vi "纳清浊度电极校准.vi"() -> ()   [LabVIEW 2016, in "斯坦道多参数.lvlib"]
uses:
  <vilib>/Utility/miscctls.llb/LVPointTypeDef.ctl
  <vilib>/Utility/miscctls.llb/LVPositionTypeDef.ctl
  <vilib>/Analysis/NI_AALBase.lvlib
  <vilib>/ptbypt/NI_PtbyPt.lvlib
panel:
  out "第三点信号值":dbl
  out "第二点信号值":dbl
  out "第一点信号值":dbl
  in  "校准量程":u16(ring) items=["0-100", "0-500", "0-2000", "0-4000"]
  in  "量程":u16(ring) items=["0-100", "0-500", "0-2000", "0-4000"]
  out "报警信息":string
  out "通讯状态":string
  out "第三点校准值":dbl
  out "标液3":sgl
  out "第二点校准值":dbl
  out "第一点校准值":dbl
  in  "校准停止":bool
  in  "校准启动":bool
  in  "校准模式":enum16{"两点校准", "单点校准", "三点校准"}(ring)=enum."单点校准"
  out "最小值":sgl format="%#.2f"
  out "最大值":sgl format="%#.2f"
  out "波形图表":dbl(graph) caption="历史曲线"
  out "mean":dbl caption="均值" format="%#.2f"
  out "standard deviation":dbl caption="标准差" format="%#.2f"
  out "变异系数":dbl format="%#.6f"
  out "测量值":sgl format="%#.2f"
  out "提示":string
  out "标液2":sgl
  out "标液1":sgl
  out "原始光强数值":u16 caption="信号值"
  out "温度":dbl format="%#.2f"
  # "浊度电极设定"
  # "℃"
  # "NTU"
  # "NTU"
  # "NTU"
  # "请选择校准模式:"
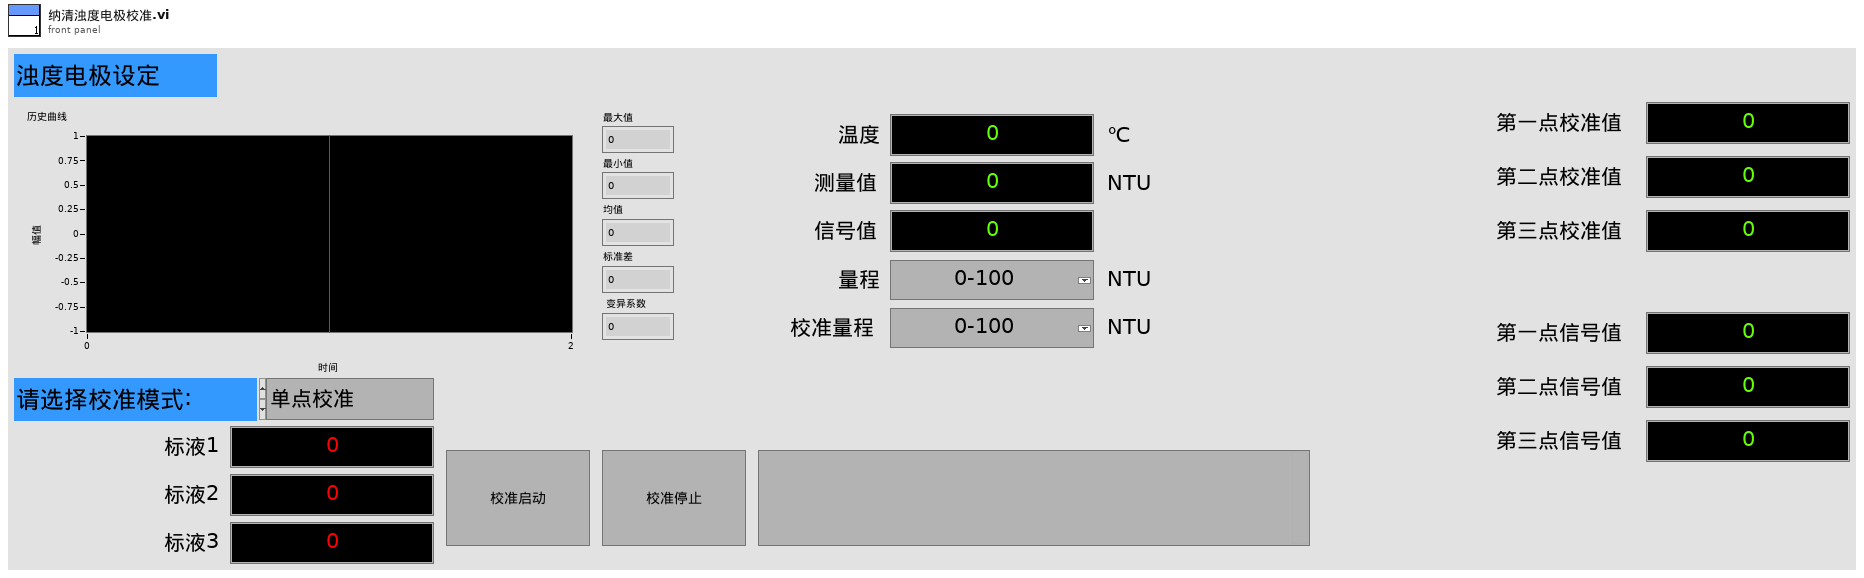
[diagram p1: front panel]
types:
  T1 = typedef "LVPointTypeDef.ctl" = cluster{"Horizontal":i16, "Vertical":i16}
  T2 = cluster{"报警码":u16, "浊度数值 NTU":sgl, "温度数据":sgl, "原始光强数值":u16, "量程":u16, "平均次数":u16, "清扫模式":u16, "清扫次数":u16, "清扫间隔分钟":u16, "0X000B_NC":string, "产品名称":string, "序列号":string, "硬件版本":string, "软件版本":string, "通讯地址":u16, "波特率":u16, "设备类型":u16, "0X0026_NC":string, "校准量程":u16, "第一点原始光强":u16, "第一点校准数据":sgl, "第二点原始光强":u16, "第二点校准数据":sgl, "第三点原始光强":u16, "第三点校准数据":sgl, "探头校准命令":u16, "温度校准参数":sgl, "温度校准命令":u16}
  T3 = typedef "LVPositionTypeDef.ctl" = cluster{"Left":i32, "Top":i32}
  T4 = enum8{"Enabled", "Disabled", "Disabled and Grayed Out"}
  T5 = cluster{"报警码":u16, "叶绿素a":sgl, "温度数据":sgl, "原始光强数值":u16, "量程":u16, "平均次数":u16, "清扫模式":u16, "清扫次数":u16, "清扫间隔分钟":u16, "0X000B_NC":string, "产品名称":string, "序列号":string, "硬件版本":string, "软件版本":string, "通讯地址":u16, "波特率":u16, "设备类型":u16, "0X0026_NC":string, "校准量程":u16, "第一点原始光强":u16, "第一点校准数据":sgl, "第二点原始光强":u16, "第二点校准数据":sgl, "第三点原始光强":u16, "第三点校准数据":sgl, "探头校准命令":u16, "温度校准参数":sgl, "温度校准命令":u16}
  T6 = cluster{"ph":bool, "DO":bool, "Cond":bool, "Turb":bool, "叶绿素a":bool, "藻密度":bool, "ORP":bool}
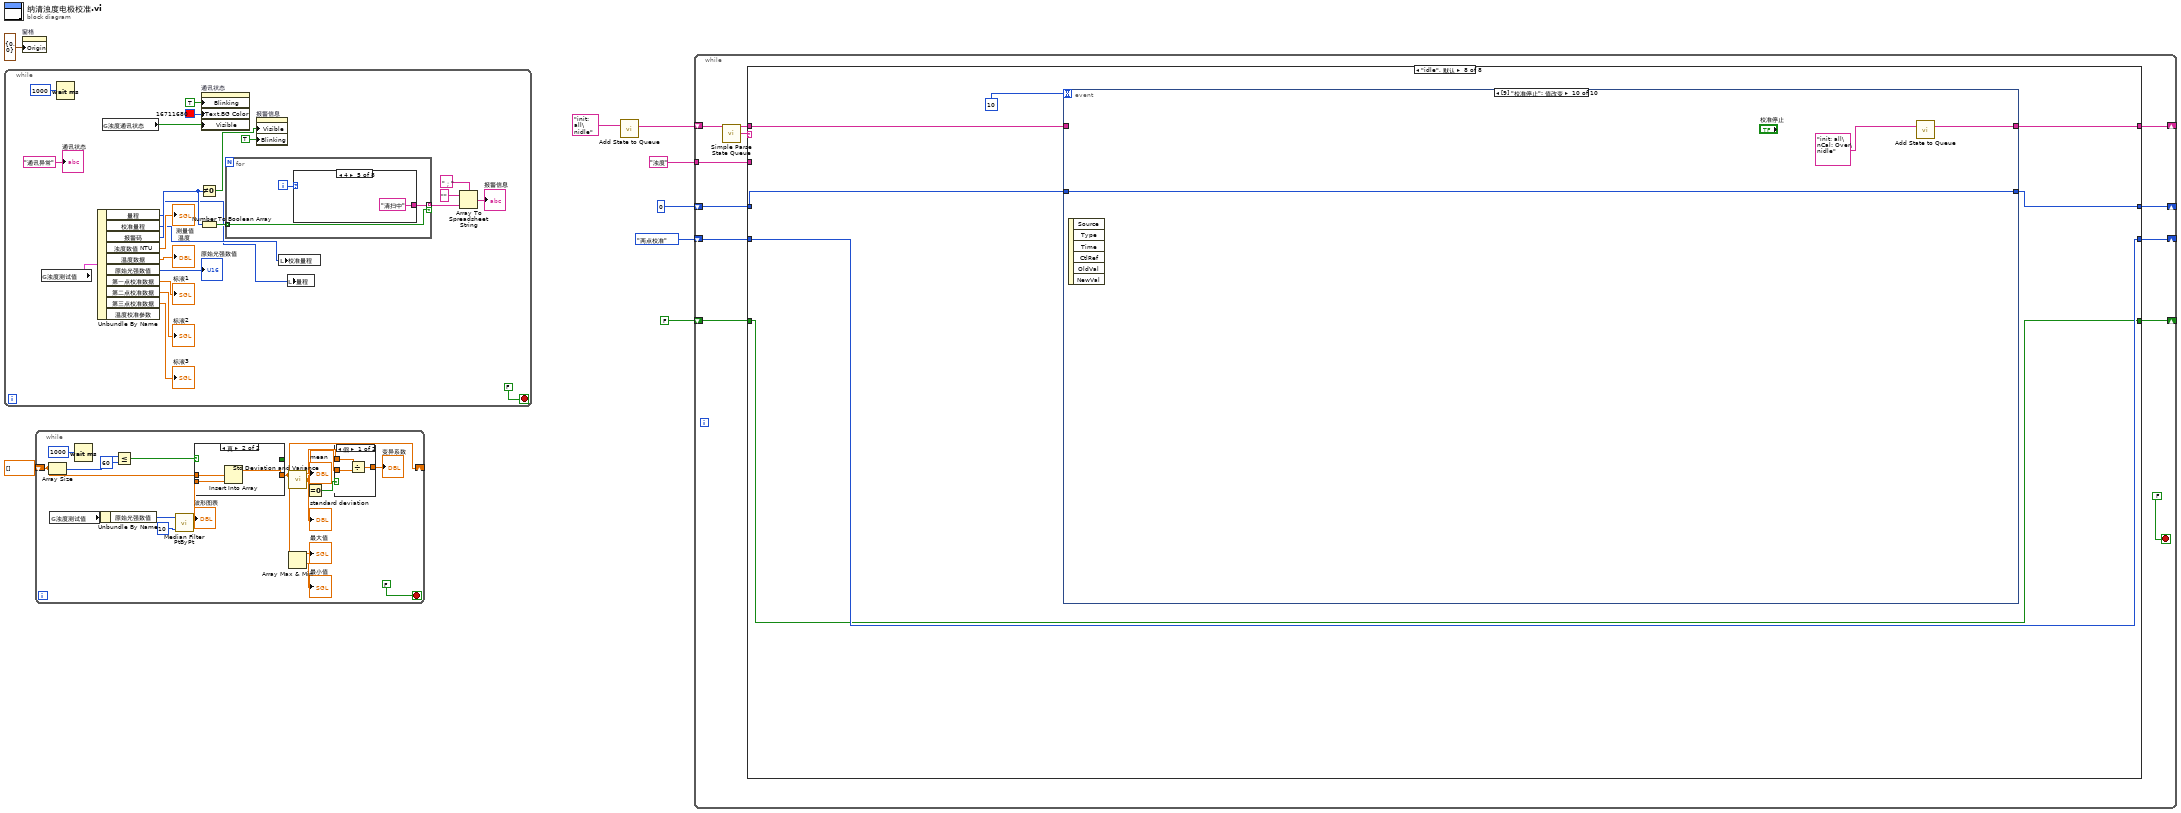
[diagram p0: block diagram]
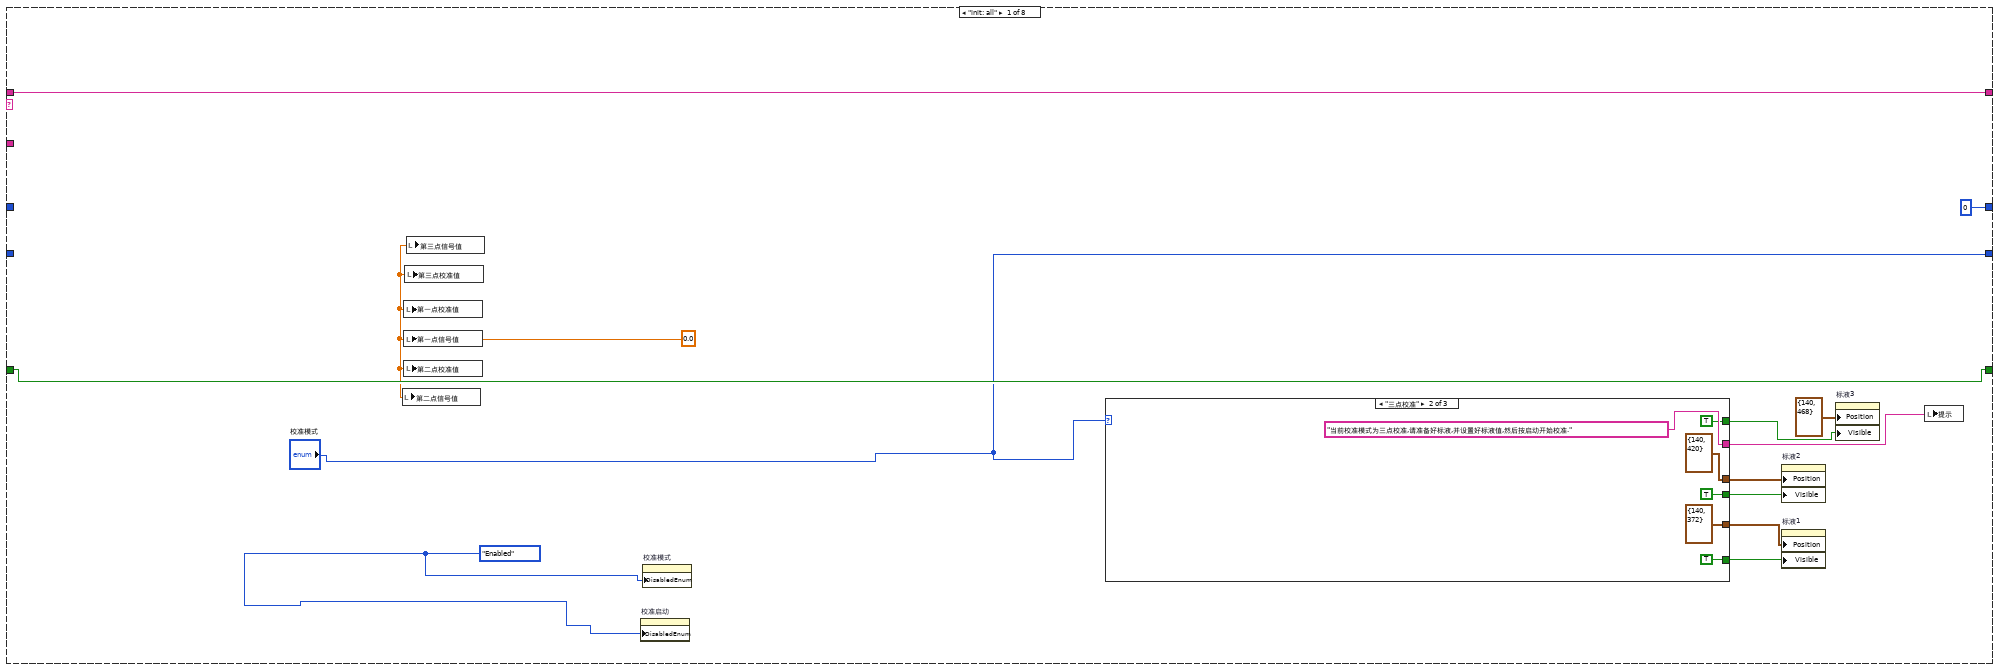
[diagram p2: hidden frame]
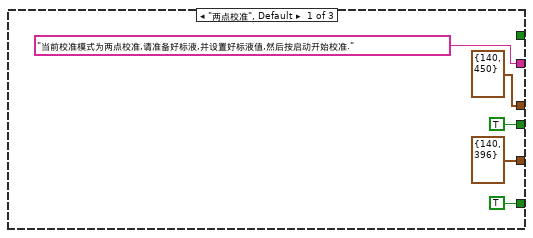
[diagram p3: hidden frame]
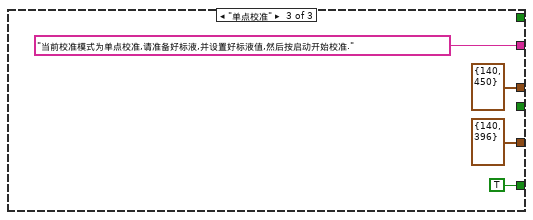
[diagram p4: hidden frame]
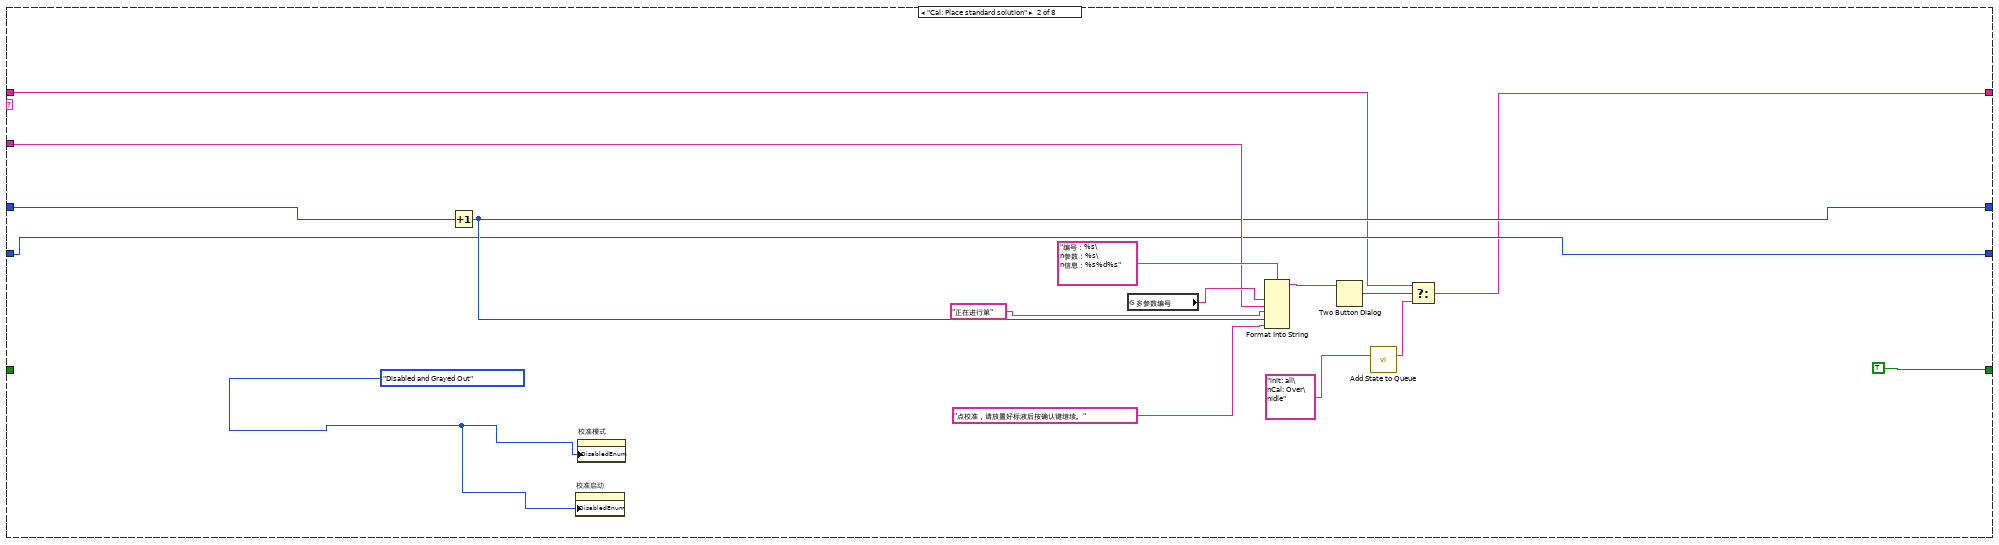
[diagram p5: hidden frame]
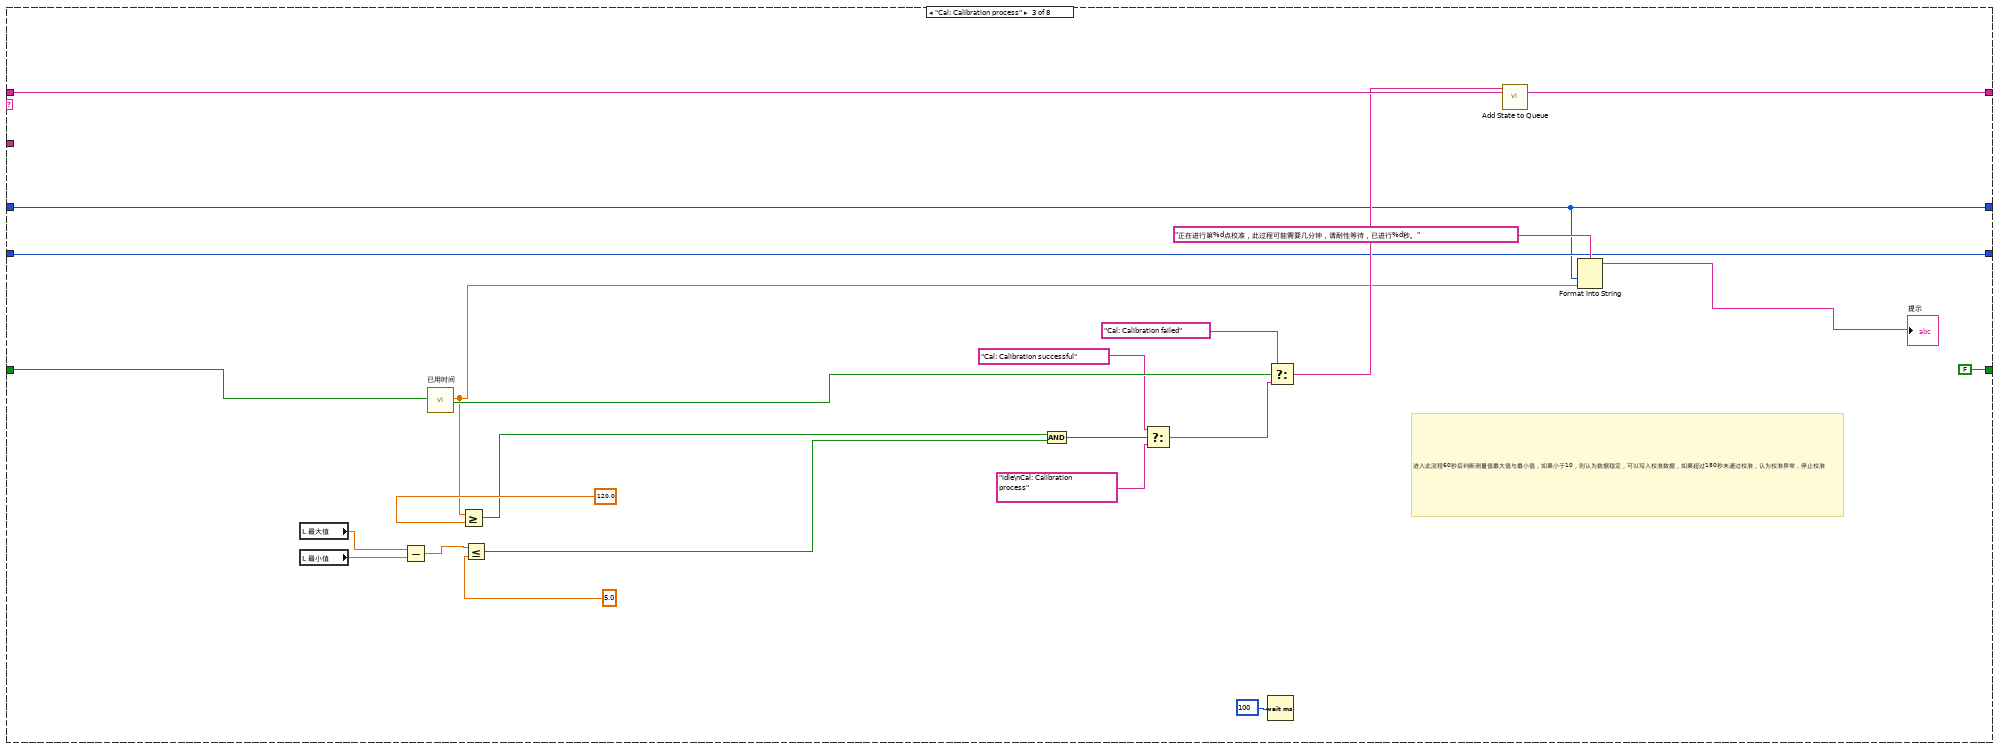
[diagram p6: hidden frame]
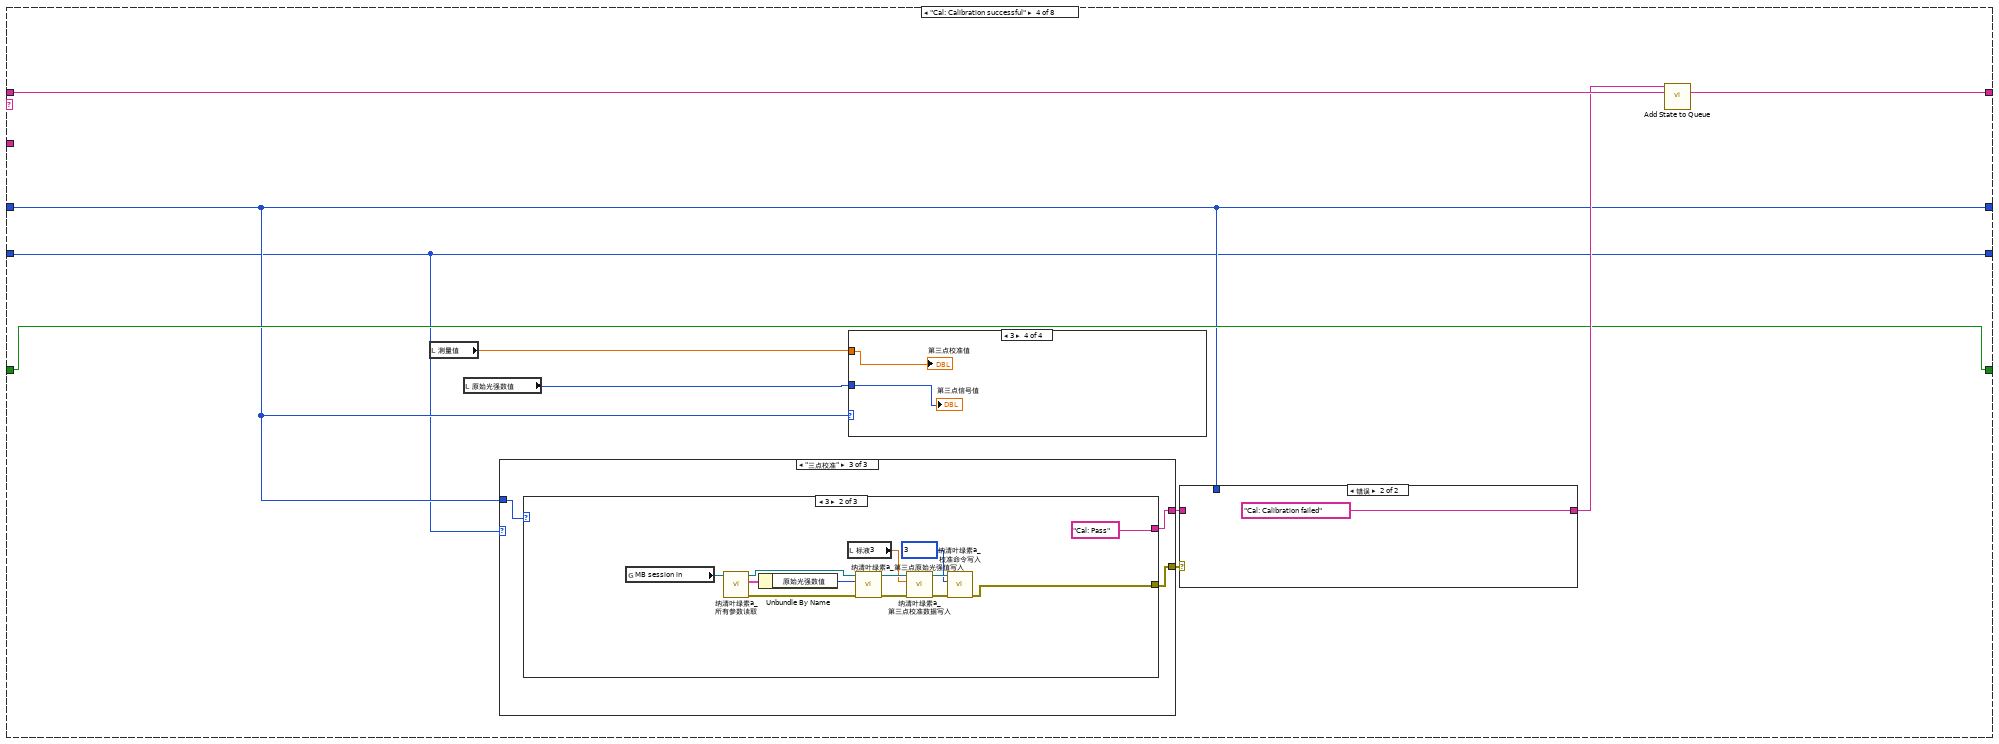
[diagram p7: hidden frame]
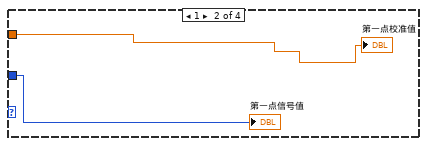
[diagram p9: hidden frame]
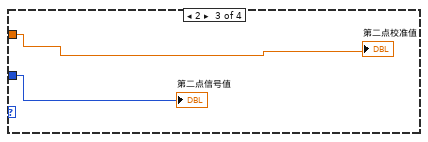
[diagram p10: hidden frame]
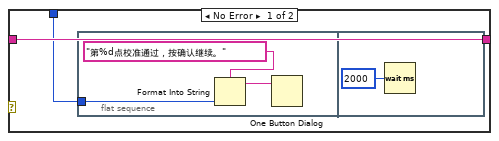
[diagram p11: hidden frame]
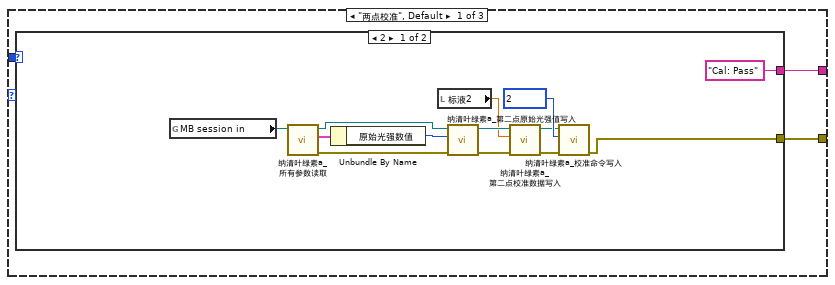
[diagram p12: hidden frame]
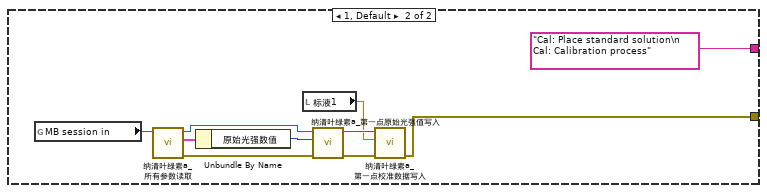
[diagram p13: hidden frame]
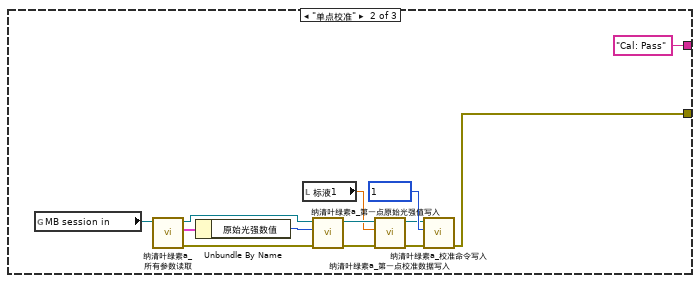
[diagram p14: hidden frame]
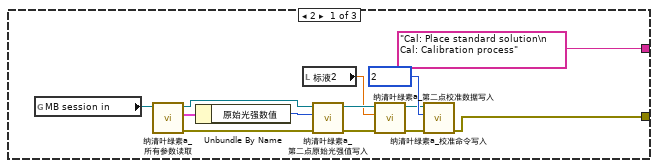
[diagram p15: hidden frame]
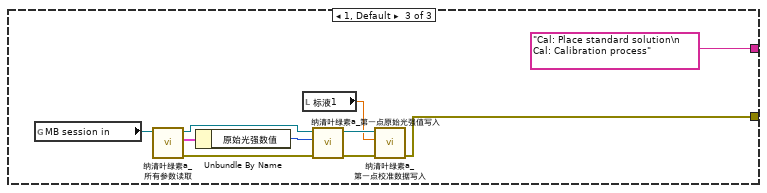
[diagram p16: hidden frame]
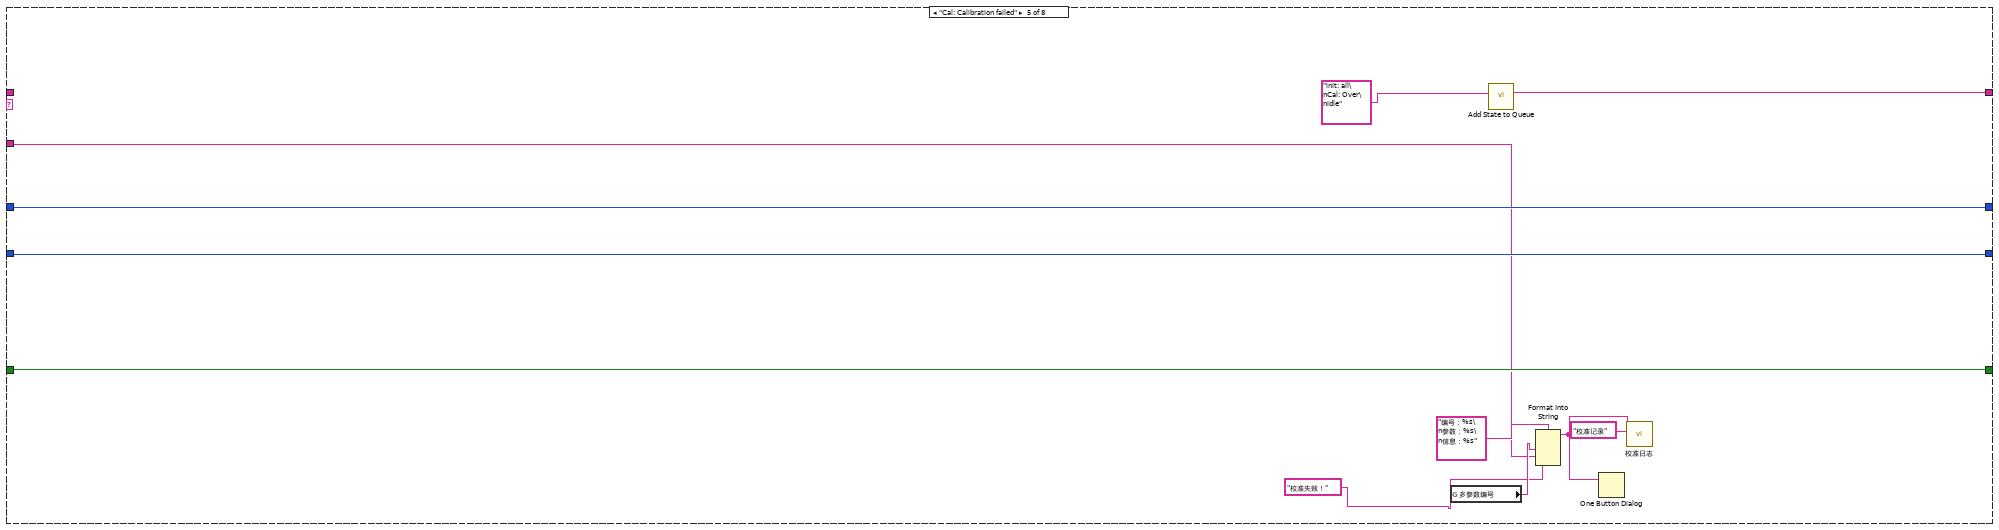
[diagram p17: hidden frame]
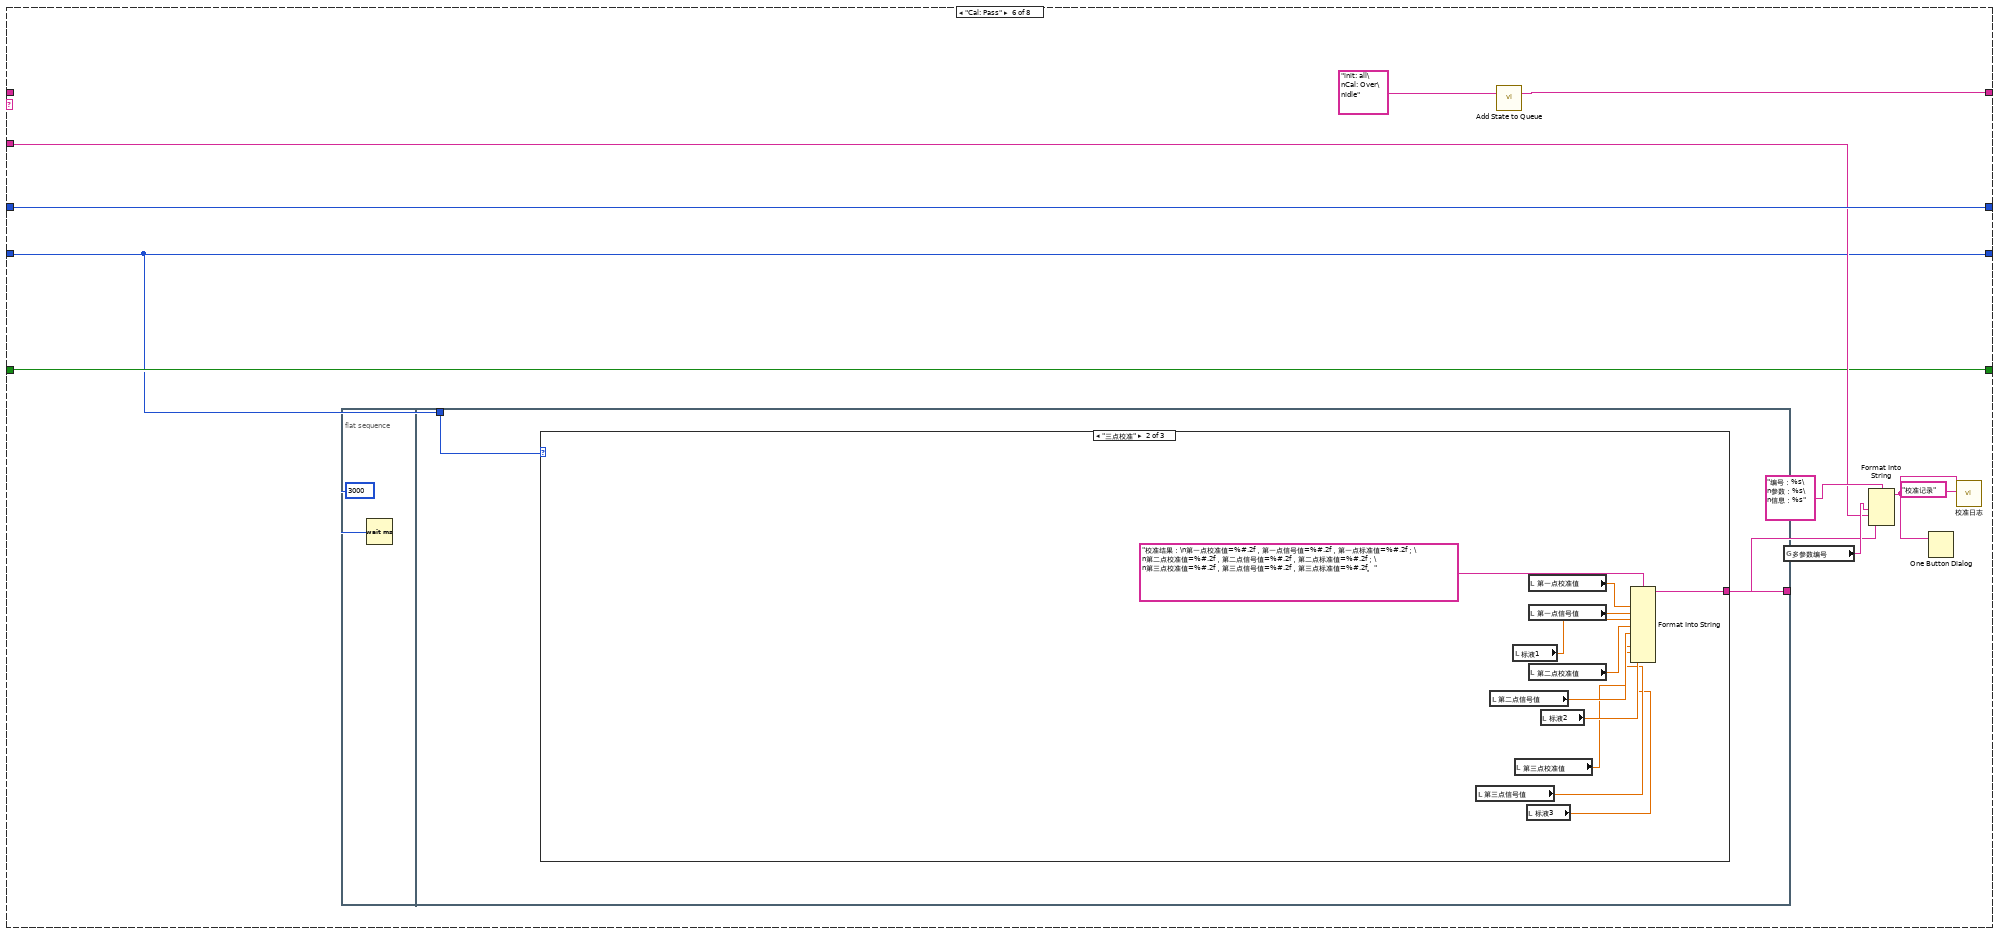
[diagram p18: hidden frame]
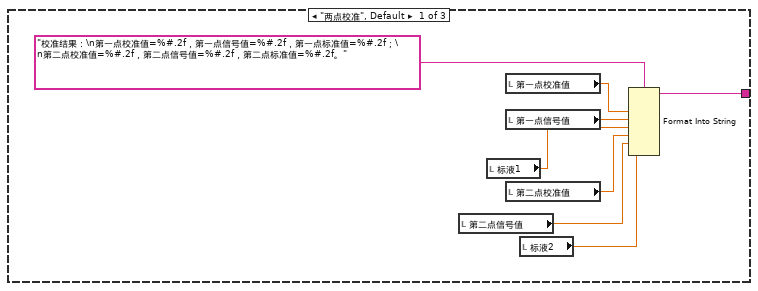
[diagram p19: hidden frame]
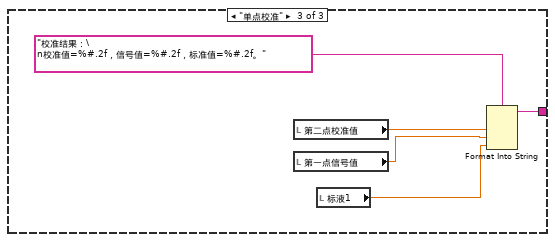
[diagram p20: hidden frame]
diagram:
  n1 = while {
    stop <- FALSE stop-if-true
    n2 = global read "纳清过程全局变量.vi" "浊度测试值"() -> (w29:T2)
    n3 = Wait (ms)(milliseconds to wait=u32 1000 ("等待时间（毫秒）")) -> ()  [unwired: 1 out]
    n4 = Unbundle By Name(w29) -> ("量程"=w9:u16, "校准量程"=w10:u16, "报警码"=w11:u16, "浊度数值 NTU"=→"测量值":sgl, "温度数据"=→"温度":sgl, "原始光强数值"=→"原始光强数值":u16, "第一点校准数据"=→"标液1":sgl, "第二点校准数据"=→"标液2":sgl, "第三点校准数据"=→"标液3":sgl)  [unwired: 1 out]
    n5 = global read "多参数全局变量.vi" "浊度通讯状态"() -> (w19:bool)
    n6 = Not Equal To 0?(x=w11) -> (x != 0?=w13:bool)
    n7 = Number To Boolean Array(number=w11) -> (Boolean array=w18:bool[])
    n8 = property on="通讯状态" class="Str"("Blinking"=TRUE ("闪烁"), "Text.BG Color"=u32 16711680, "Visible"=w19) -> ()  [unwired: 2 in, 2 out]
    n9 = for {
      tunnel: w18 -> [w32] mode=indexing
      tunnel: [w33] -> w17 mode=indexing if=w32
      i -> [w34]
      n10 = case shown="4" w34 {
        tunnel: [_ "浊度超量程" "温度超量程" "光强信号超范围" "清扫中" "温度传感器故障" "电极故障" "内部电压基准故障"] -> w33
        frame Default {
        }
        frame 0 {
        }
        frame 2 {
        }
        frame 3 {
        }
        frame 4 {
        }
        frame 8 {
        }
        frame 9 {
        }
        frame 10 {
        }
      }
    }
    n11 = property on="报警信息" class="Str"("Visible"=w13, "Blinking"=TRUE ("闪烁")) -> ()  [unwired: 2 in, 2 out]
    n12 = local write "校准量程"(w10) -> ()
    n13 = local write "量程"(w9) -> ()
    n14 = Array To Spreadsheet String(delimiter (Tab)="；" ("分隔符(Tab)"), array=w17, 3:"" ("格式字符串")) -> (spreadsheet string=→"报警信息":string)
    "通讯状态" <- "通讯异常" ("当前串口")
  }
  n15 = property on="窗格" class="Pane"("Origin"=T1 {"Horizontal"=0, "Vertical"=0} ("原点")) -> ()  [unwired: 2 in, 2 out]
  n16 = while {
    shift-right: [w48] -> _
    shift-left: sgl[] [] -> [w54]
    stop <- FALSE stop-if-true
    n17 = Array Size(array=w54) -> (size(s)=w56:i32)
    n18 = global read "纳清过程全局变量.vi" "浊度测试值"() -> (w45:T2)
    n19 = Wait (ms)(milliseconds to wait=u32 1000 ("等待时间（毫秒）")) -> ()  [unwired: 1 out]
    n20 = Unbundle By Name(w45) -> ("原始光强数值"=w43:u16)
    n21 = Less Or Equal?(x=w56, y=60) -> (x <= y?=w55:bool)
    n22 = call <vilib>:"Median Filter PtByPt.vi"("rank"=10, "x"=w43) -> ("Filtered x"=w42:dbl)  [unwired: 2 in, 1 out]
    "波形图表" <- w42
    n23 = case shown="真" w55 {
      tunnel: w54 -> [w67 w70]
      tunnel: w42 -> [w65 w69]
      tunnel: [w63 w68] -> w48
      tunnel: [TRUE _] -> _
      frame False {
        n24 = Replace Array Subset(array=w67, new element=w65) -> (w66:sgl[])  [unwired: 1 in]
        n25 = Rotate 1D Array(1:w66, 2:-1 ("n")) -> (0:w63:sgl[])
      }
      frame True {
        n26 = Insert Into Array(array=w70, new element=w69) -> (w68:sgl[])  [unwired: 1 in]
      }
    }
    n27 = call <vilib>:"Std Deviation and Variance.vi"("X"=w48) -> ("mean"=w52:dbl, "standard deviation"=w51:dbl)  [unwired: 1 in, 1 out]
    "mean" <- w52
    "standard deviation" <- w51
    n28 = Array Max & Min(array=w48) -> (max value=→"最大值":sgl, min value=→"最小值":sgl)  [unwired: 2 out]
    n29 = Equal To 0?(x=w52) -> (x = 0?=w53:bool)
    n30 = case shown="假" w53 {
      tunnel: w51 -> [w61 _]
      tunnel: [w60 _] -> w50
      tunnel: w52 -> [w59 _]
      frame False {
        n31 = Divide(x=w61, y=w59) -> (x/y=w60:dbl)
      }
      frame True {
      }
    }
    "变异系数" <- w50
  }
  n32 = call "Add State to Queue.vi"("State(s) In (\"\")"="init: all\nidle" ("State(s) In (\"\")")) -> ("States Out"=w5:string)  [unwired: 14 in]
  n33 = while {
    shift-right: [w78] -> _
    shift-left: w5 -> [w82]
    shift-right: [w75] -> _
    shift-left: 0 -> [w77]
    tunnel: "浊度" ("State(s) In (\"\")") -> [w76]
    shift-right: [w73] -> _
    shift-left: enum16{"两点校准", "单点校准", "三点校准"}."两点校准" ("校准模式") -> [w74]
    shift-right: [w71] -> _
    shift-left: FALSE -> [w72]
    stop <- FALSE stop-if-true
    n34 = call "Simple Parse State Queue.vi"("State Queue"=w82) -> ("Remain States"=w79:string, "Next State"=w80:string)  [unwired: 13 in]
    n35 = case shown="\"idle\", 默认" w80 {
      tunnel: w79 -> [w95 w114 w145 w158 _ _ w307 w314]
      tunnel: [w95 w113 w144 w157 w259 w264 w307 w313] -> w78
      tunnel: w77 -> [_ w122 w129 w152 w262 w273 w306 w311]
      tunnel: w76 -> [_ w123 _ _ w253 w269 _ _]
      tunnel: [0 w120 w129 w152 w262 w273 w306 w312] -> w75
      tunnel: w74 -> [_ w119 w130 w151 w261 w265 w305 w310]
      tunnel: ["校准模式" w119 w130 w151 w261 w265 w305 w310] -> w73
      tunnel: w72 -> [w93 _ w132 w153 w260 w268 w304 w308]
      tunnel: [w93 TRUE FALSE w153 w260 w268 w304 w308] -> w71
      frame "init: all" {
        w91 = T4."Enabled" ("禁用")
        w92 = 0.0 ("第一点校准值")
        n36 = local write "第二点信号值"(w92) -> ()
        n37 = local write "第一点校准值"(w92) -> ()
        n38 = local write "第一点信号值"(w92) -> ()
        n39 = local write "第二点校准值"(w92) -> ()
        n40 = local write "第三点校准值"(w92) -> ()
        n41 = local write "第三点信号值"(w92) -> ()
        n42 = property on="校准启动" class="Bool"("DisabledEnum"=w91) -> ()  [unwired: 2 in, 2 out]
        n43 = property on="校准模式" class="Enum (严格)"("DisabledEnum"=w91) -> ()  [unwired: 2 in, 2 out]
        n44 = case shown="\"三点校准\"" "校准模式" {
          tunnel: ["当前校准模式为两点校准,请准备好标液,并设置好标液值,然后按启动开始校准." ("提示") "当前校准模式为三点校准,请准备好标液,并设置好标液值,然后按启动开始校准." ("提示") "当前校准模式为单点校准,请准备好标液,并设置好标液值,然后按启动开始校准." ("提示")] -> w83
          tunnel: [TRUE ("可见") TRUE ("可见") _] -> w88
          tunnel: [T3 {"Left"=140, "Top"=396} ("位置") T3 {"Left"=140, "Top"=372} ("位置") T3 {"Left"=140, "Top"=396} ("位置")] -> w85
          tunnel: [T3 {"Left"=140, "Top"=450} ("位置 2") T3 {"Left"=140, "Top"=420} ("位置 2") T3 {"Left"=140, "Top"=450} ("位置 2")] -> w86
          tunnel: [_ TRUE ("可见") _] -> w89
          tunnel: [TRUE ("可见") TRUE ("可见") TRUE ("可见")] -> w90
          frame "两点校准", Default {
          }
          frame "三点校准" {
          }
          frame "单点校准" {
          }
        }
        n45 = property on="标液2" class="DigNum (严格)"("Position"=w86, "Visible"=w88) -> ()  [unwired: 2 in, 2 out]
        n46 = property on="标液1" class="DigNum (严格)"("Position"=w85, "Visible"=w90) -> ()  [unwired: 2 in, 2 out]
        n47 = property on="标液3" class="DigNum (严格)"("Position"=T3 {"Left"=140, "Top"=468} ("位置 3"), "Visible"=w89) -> ()  [unwired: 2 in, 2 out]
        n48 = local write "提示"(w83) -> ()
      }
      frame "Cal: Place standard solution" {
        w112 = T4."Disabled and Grayed Out" ("禁用")
        n49 = Increment(x=w122) -> (x+1=w120:i32)
        n50 = property on="校准启动" class="Bool"("DisabledEnum"=w112) -> ()  [unwired: 2 in, 2 out]
        n51 = property on="校准模式" class="Enum (严格)"("DisabledEnum"=w112) -> ()  [unwired: 2 in, 2 out]
        n52 = global read "多参数全局变量.vi" "多参数编号"() -> (w125:string)
        n53 = Format Into String(format string="编号：%s\n参数：%s\n信息：%s%d%s" ("格式字符串"), w125, w123, "正在进行第" ("消息"), w120, "点校准，请放置好标液后按确认键继续。" ("消息")) -> (resulting string=w117:string)  [unwired: 2 in, 1 out]
        n54 = Two Button Dialog(message=w117) -> (T button?=w116:bool)  [unwired: 2 in]
        n55 = call "Add State to Queue.vi"("State(s) In (\"\")"="init: all\nCal: Over\nidle" ("State(s) In (\"\")")) -> ("States Out"=w115:string)  [unwired: 14 in]
        n56 = Select(t=w114, s=w116, f=w115) -> (s? t:f=w113:string)
      }
      frame "Cal: Calibration process" {
        # "进入此流程60秒后判断测量值最大值与最小值，如果小于10，则认为数据稳定，可以写入校准数据，如果超过180秒未通过校准，认为校准异常，停止校准"
        n57 = local read "最大值"() -> (w149:sgl)
        n58 = local read "最小值"() -> (w148:sgl)
        n59 = Subtract(x=w149, y=w148) -> (x-y=w150:sgl)
        n60 = call "已用时间"("Reset"=w132) -> ("Elapsed Time (s)"=w128:dbl, "Time has Elapsed"=w146:bool)  [unwired: 11 in, 6 out]
        n61 = Greater Or Equal?(x=w128, y=120.0) -> (x >= y?=w141:bool)
        n62 = Less Or Equal?(x=w150, y=5.0) -> (x <= y?=w137:bool)
        n63 = And(x=w141, y=w137) -> (x .and. y?=w138:bool)
        n64 = Select(t="Cal: Calibration successful" ("State(s) In (\"\")"), s=w138, f="idle\nCal: Calibration process" ("State(s) In (\"\")")) -> (s? t:f=w136:string)
        n65 = Wait (ms)(milliseconds to wait=u32 100 ("等待时间（毫秒）")) -> ()  [unwired: 1 out]
        n66 = Select(t="Cal: Calibration failed" ("State(s) In (\"\")"), s=w146, f=w136) -> (s? t:f=w135:string)
        n67 = call "Add State to Queue.vi"("State(s) In Front (\"\")"=w135, "State(s) In (\"\")"=w145) -> ("States Out"=w144:string)  [unwired: 13 in]
        n68 = Format Into String(format string="正在进行第%d点校准，此过程可能需要几分钟，请耐性等待，已进行%d秒。" ("格式字符串"), w129, w128) -> (resulting string=→"提示":string)  [unwired: 2 in, 1 out]
      }
      frame "Cal: Calibration successful" {
        n69 = local read "测量值"() -> (w154:sgl)
        n70 = local read "原始光强数值"() -> (w155:u16)
        n71 = case shown="\"三点校准\"" w151 {
          tunnel: [w176 w200 w213] -> w160
          tunnel: [w175 "Cal: Pass" ("State(s) In (\"\")") w214] -> w159
          tunnel: w152 -> [w174 _ w215]
          frame "两点校准", Default {
            n72 = case shown="2" w174 {
              tunnel: [w177 w190] -> w176
              tunnel: ["Cal: Pass" ("State(s) In (\"\")") "Cal: Place standard solution\n Cal: Calibration process" ("State(s) In (\"\")")] -> w175
              frame 2 {
                n73 = global read "多参数全局变量.vi" "MB session in"() -> (w185:refnum<class "MB_Master.lvclass">)
                n74 = call "纳清叶绿素a_所有参数读取.vi"("MB session in"=w185) -> ("error out"=w187:errorcluster, "输出值"=w184:T5, "MB session out"=w186:refnum<class "MB_Master.lvclass">)  [unwired: 8 in]
                n75 = Unbundle By Name(w184) -> ("原始光强数值"=w183:u16)
                n76 = local read "标液2"() -> (w178:sgl)
                n77 = call "纳清叶绿素a_第二点原始光强值写入.vi"("error in (no error)"=w187, "数值"=w183, "MB session in"=w186) -> ("error out"=w182:errorcluster, "MB session out"=w181:refnum<class "MB_Master.lvclass">)  [unwired: 7 in]
                n78 = call "纳清叶绿素a_第二点校准数据写入.vi"("error in (no error)"=w182, "数值"=w178, "MB session in"=w181) -> ("error out"=w180:errorcluster, "MB session out"=w179:refnum<class "MB_Master.lvclass">)  [unwired: 7 in]
                n79 = call "纳清叶绿素a_校准命令写入.vi"("error in (no error)"=w180, "数值"=u16 2 ("starting address"), "MB session in"=w179) -> ("error out"=w177:errorcluster)  [unwired: 7 in, 1 out]
              }
              frame 1, Default {
                n80 = global read "多参数全局变量.vi" "MB session in"() -> (w196:refnum<class "MB_Master.lvclass">)
                n81 = call "纳清叶绿素a_所有参数读取.vi"("MB session in"=w196) -> ("error out"=w198:errorcluster, "输出值"=w195:T5, "MB session out"=w197:refnum<class "MB_Master.lvclass">)  [unwired: 8 in]
                n82 = Unbundle By Name(w195) -> ("原始光强数值"=w194:u16)
                n83 = local read "标液1"() -> (w191:sgl)
                n84 = call "纳清叶绿素a_第一点原始光强值写入.vi"("error in (no error)"=w198, "数值"=w194, "MB session in"=w197) -> ("error out"=w193:errorcluster, "MB session out"=w192:refnum<class "MB_Master.lvclass">)  [unwired: 7 in]
                n85 = call "纳清叶绿素a_第一点校准数据写入.vi"("error in (no error)"=w193, "数值"=w191, "MB session in"=w192) -> ("error out"=w190:errorcluster)  [unwired: 7 in, 1 out]
              }
            }
          }
          frame "单点校准" {
            n86 = global read "多参数全局变量.vi" "MB session in"() -> (w208:refnum<class "MB_Master.lvclass">)
            n87 = call "纳清叶绿素a_所有参数读取.vi"("MB session in"=w208) -> ("error out"=w210:errorcluster, "输出值"=w207:T5, "MB session out"=w209:refnum<class "MB_Master.lvclass">)  [unwired: 8 in]
            n88 = Unbundle By Name(w207) -> ("原始光强数值"=w206:u16)
            n89 = local read "标液1"() -> (w201:sgl)
            n90 = call "纳清叶绿素a_第一点原始光强值写入.vi"("error in (no error)"=w210, "数值"=w206, "MB session in"=w209) -> ("error out"=w205:errorcluster, "MB session out"=w204:refnum<class "MB_Master.lvclass">)  [unwired: 7 in]
            n91 = call "纳清叶绿素a_第一点校准数据写入.vi"("error in (no error)"=w205, "数值"=w201, "MB session in"=w204) -> ("error out"=w203:errorcluster, "MB session out"=w202:refnum<class "MB_Master.lvclass">)  [unwired: 7 in]
            n92 = call "纳清叶绿素a_校准命令写入.vi"("error in (no error)"=w203, "数值"=u16 1 ("starting address"), "MB session in"=w202) -> ("error out"=w200:errorcluster)  [unwired: 7 in, 1 out]
          }
          frame "三点校准" {
            n93 = case shown="3" w215 {
              tunnel: [w217 w229 w242] -> w213
              tunnel: ["Cal: Place standard solution\n Cal: Calibration process" ("State(s) In (\"\")") "Cal: Pass" ("State(s) In (\"\")") "Cal: Place standard solution\n Cal: Calibration process" ("State(s) In (\"\")")] -> w214
              frame 2 {
                n94 = global read "多参数全局变量.vi" "MB session in"() -> (w225:refnum<class "MB_Master.lvclass">)
                n95 = call "纳清叶绿素a_所有参数读取.vi"("MB session in"=w225) -> ("error out"=w227:errorcluster, "输出值"=w224:T5, "MB session out"=w226:refnum<class "MB_Master.lvclass">)  [unwired: 8 in]
                n96 = Unbundle By Name(w224) -> ("原始光强数值"=w223:u16)
                n97 = local read "标液2"() -> (w218:sgl)
                n98 = call "纳清叶绿素a_第二点原始光强值写入.vi"("error in (no error)"=w227, "数值"=w223, "MB session in"=w226) -> ("error out"=w222:errorcluster, "MB session out"=w221:refnum<class "MB_Master.lvclass">)  [unwired: 7 in]
                n99 = call "纳清叶绿素a_第二点校准数据写入.vi"("error in (no error)"=w222, "数值"=w218, "MB session in"=w221) -> ("error out"=w220:errorcluster, "MB session out"=w219:refnum<class "MB_Master.lvclass">)  [unwired: 7 in]
                n100 = call "纳清叶绿素a_校准命令写入.vi"("error in (no error)"=w220, "数值"=u16 2 ("starting address"), "MB session in"=w219) -> ("error out"=w217:errorcluster)  [unwired: 7 in, 1 out]
              }
              frame 3 {
                n101 = global read "多参数全局变量.vi" "MB session in"() -> (w238:refnum<class "MB_Master.lvclass">)
                n102 = call "纳清叶绿素a_所有参数读取.vi"("MB session in"=w238) -> ("error out"=w240:errorcluster, "输出值"=w237:T5, "MB session out"=w239:refnum<class "MB_Master.lvclass">)  [unwired: 8 in]
                n103 = Unbundle By Name(w237) -> ("原始光强数值"=w236:u16)
                n104 = local read "标液3"() -> (w230:sgl)
                n105 = call "纳清叶绿素a_第三点原始光强值写入.vi"("error in (no error)"=w240, "数值"=w236, "MB session in"=w239) -> ("error out"=w235:errorcluster, "MB session out"=w234:refnum<class "MB_Master.lvclass">)  [unwired: 7 in]
                n106 = call "纳清叶绿素a_第三点校准数据写入.vi"("error in (no error)"=w235, "数值"=w230, "MB session in"=w234) -> ("error out"=w233:errorcluster, "MB session out"=w232:refnum<class "MB_Master.lvclass">)  [unwired: 7 in]
                n107 = call "纳清叶绿素a_校准命令写入.vi"("error in (no error)"=w233, "数值"=u16 3 ("starting address"), "MB session in"=w232) -> ("error out"=w229:errorcluster)  [unwired: 7 in, 1 out]
              }
              frame 1, Default {
                n108 = global read "多参数全局变量.vi" "MB session in"() -> (w248:refnum<class "MB_Master.lvclass">)
                n109 = call "纳清叶绿素a_所有参数读取.vi"("MB session in"=w248) -> ("error out"=w250:errorcluster, "输出值"=w247:T5, "MB session out"=w249:refnum<class "MB_Master.lvclass">)  [unwired: 8 in]
                n110 = Unbundle By Name(w247) -> ("原始光强数值"=w246:u16)
                n111 = local read "标液1"() -> (w243:sgl)
                n112 = call "纳清叶绿素a_第一点原始光强值写入.vi"("error in (no error)"=w250, "数值"=w246, "MB session in"=w249) -> ("error out"=w245:errorcluster, "MB session out"=w244:refnum<class "MB_Master.lvclass">)  [unwired: 7 in]
                n113 = call "纳清叶绿素a_第一点校准数据写入.vi"("error in (no error)"=w245, "数值"=w243, "MB session in"=w244) -> ("error out"=w242:errorcluster)  [unwired: 7 in, 1 out]
              }
            }
          }
        }
        n114 = case shown="3" w152 {
          tunnel: w155 -> [_ w162 w164 w165]
          tunnel: w154 -> [_ w161 w163 w166]
          frame 0, Default {
          }
          frame 1 {
            "第一点信号值" <- w162
            "第一点校准值" <- w161
          }
          frame 2 {
            "第二点信号值" <- w164
            "第二点校准值" <- w163
          }
          frame 3 {
            "第三点校准值" <- w166
            "第三点信号值" <- w165
          }
        }
        n115 = case shown="错误" w160 {
          tunnel: w159 -> [w168 _]
          tunnel: [w168 "Cal: Calibration failed" ("State(s) In (\"\")")] -> w156
          tunnel: w152 -> [w167 _]
          frame No Error {
            n116 = flat-sequence {
              tunnel: w167 -> [w169]
              frame #0 {
                n117 = Format Into String(format string="第%d点校准通过，按确认继续。" ("格式字符串"), w169) -> (resulting string=w171:string)  [unwired: 2 in, 1 out]
                n118 = One Button Dialog(message=w171) -> ()  [unwired: 1 in, 1 out]
              }
              frame #1 {
                n119 = Wait (ms)(milliseconds to wait=u32 2000 ("等待时间（毫秒）")) -> ()  [unwired: 1 out]
              }
            }
          }
          frame Error {
          }
        }
        n120 = call "Add State to Queue.vi"("State(s) In Front (\"\")"=w156, "State(s) In (\"\")"=w158) -> ("States Out"=w157:string)  [unwired: 13 in]
      }
      frame "Cal: Calibration failed" {
        n121 = global read "多参数全局变量.vi" "多参数编号"() -> (w256:string)
        n122 = call "Add State to Queue.vi"("State(s) In (\"\")"="init: all\nCal: Over\nidle" ("State(s) In (\"\")")) -> ("States Out"=w259:string)  [unwired: 14 in]
        n123 = Format Into String(format string="编号：%s\n参数：%s\n信息：%s" ("格式字符串"), w256, w253, "校准失败！" ("消息")) -> (resulting string=w255:string)  [unwired: 2 in, 1 out]
        n124 = One Button Dialog(message=w255) -> ()  [unwired: 1 in, 1 out]
        n125 = call "校准日志.vi"("table"="校准记录", "日志信息"=w255) -> ()  [unwired: 9 in, 1 out]
      }
      frame "Cal: Pass" {
        n126 = flat-sequence {
          tunnel: [w276] -> w266
          tunnel: w265 -> [w275]
          frame #0 {
            n127 = Wait (ms)(milliseconds to wait=u32 3000 ("等待时间（毫秒）")) -> ()  [unwired: 1 out]
          }
          frame #1 {
            n128 = case shown="\"三点校准\"" w275 {
              tunnel: [w284 w295 w300] -> w276
              frame "两点校准", Default {
                n129 = local read "第二点信号值"() -> (w278:dbl)
                n130 = local read "标液1"() -> (w280:sgl)
                n131 = local read "第一点校准值"() -> (w282:dbl)
                n132 = local read "第一点信号值"() -> (w283:dbl)
                n133 = local read "第二点校准值"() -> (w279:dbl)
                n134 = local read "标液2"() -> (w277:sgl)
                n135 = Format Into String(format string="校准结果：\n第一点校准值=%#.2f，第一点信号值=%#.2f，第一点标准值=%#.2f；\n第二点校准值=%#.2f，第二点信号值=%#.2f，第二点标准值=%#.2f。" ("提示"), w282, w283, w280, w279, w278, w277) -> (resulting string=w284:string)  [unwired: 2 in, 1 out]
              }
              frame "三点校准" {
                n136 = local read "第三点信号值"() -> (w286:dbl)
                n137 = local read "第二点信号值"() -> (w289:dbl)
                n138 = local read "标液1"() -> (w291:sgl)
                n139 = local read "第三点校准值"() -> (w287:dbl)
                n140 = local read "标液3"() -> (w285:sgl)
                n141 = local read "第一点校准值"() -> (w293:dbl)
                n142 = local read "第一点信号值"() -> (w294:dbl)
                n143 = local read "第二点校准值"() -> (w290:dbl)
                n144 = local read "标液2"() -> (w288:sgl)
                n145 = Format Into String(format string="校准结果：\n第一点校准值=%#.2f，第一点信号值=%#.2f，第一点标准值=%#.2f；\n第二点校准值=%#.2f，第二点信号值=%#.2f，第二点标准值=%#.2f；\n第三点校准值=%#.2f，第三点信号值=%#.2f，第三点标准值=%#.2f。" ("提示"), w293, w294, w291, w290, w289, w288, w287, w286, w285) -> (resulting string=w295:string)  [unwired: 2 in, 1 out]
              }
              frame "单点校准" {
                n146 = local read "第二点校准值"() -> (w299:dbl)
                n147 = local read "第一点信号值"() -> (w297:dbl)
                n148 = local read "标液1"() -> (w296:sgl)
                n149 = Format Into String(format string="校准结果：\n校准值=%#.2f，信号值=%#.2f，标准值=%#.2f。" ("提示"), w299, w297, w296) -> (resulting string=w300:string)  [unwired: 2 in, 1 out]
              }
            }
          }
        }
        n150 = call "Add State to Queue.vi"("State(s) In (\"\")"="init: all\nCal: Over\nidle" ("State(s) In (\"\")")) -> ("States Out"=w264:string)  [unwired: 14 in]
        n151 = global read "多参数全局变量.vi" "多参数编号"() -> (w270:string)
        n152 = Format Into String(format string="编号：%s\n参数：%s\n信息：%s" ("格式字符串"), w270, w269, w266) -> (resulting string=w267:string)  [unwired: 2 in, 1 out]
        n153 = One Button Dialog(message=w267) -> ()  [unwired: 1 in, 1 out]
        n154 = call "校准日志.vi"("table"="校准记录", "日志信息"=w267) -> ()  [unwired: 9 in, 1 out]
      }
      frame "Cal: Over" {
        n155 = global read "多参数全局变量.vi" "校准运行状态"() -> (w302:T6)
        n156 = Bundle By Name(cluster=w302, "Turb"=FALSE ("Cond")) -> (w303:T6)
        n157 = global write "多参数全局变量.vi" "校准运行状态"(w303) -> ()
      }
      frame "idle", Default {
        n158 = event shown="[9] \"校准停止\": 值改变" {
          selector: _ -> [_ _ _ _ _ _ _ _ _ _]
          dyn-events: _ -> [_ _ _ _ _ _ _ _ _ _]
          timeout: 10 -> [_ _ _ _ _ _ _ _ _ _]
          tunnel: w314 -> [w317 w321 w324 w331 w336 w341 w346 w351 w362 _]
          tunnel: [w316 w320 w325 w335 w340 w345 w350 w355 w361 w364] -> w313
          tunnel: [w315 w318 w326 w334 w339 w344 w349 w354 w359 w365] -> w312
          tunnel: w311 -> [w315 w318 w326 w334 w339 w344 w349 w354 w359 w365]
          event Timeout {
            n159 = event-data() -> ()  [unwired: 1 in, 3 out]
            n160 = call "Add State to Queue.vi"("State(s) In (\"\")"=w317) -> ("States Out"=w316:string)  [unwired: 14 in]
          }
          event "校准模式": Value Change {
            n161 = event-data() -> ()  [unwired: 1 in, 6 out]
            n162 = call "Add State to Queue.vi"("State(s) In (\"\")"=w321, "State(s) At Back (\"\")"="init: all\nidle" ("State(s) In (\"\")")) -> ("States Out"=w320:string)  [unwired: 13 in]
          }
          event "标液1", "标液2", "标液3": Mouse Down {
            n163 = event-data() -> ("CtlRef"=w323:refnum<vi>)  [unwired: 1 in, 7 out]
            n164 = property class="DigNum (严格)"(reference=w323) -> ("DisabledEnum"=w322:T4)  [unwired: 1 in, 2 out]
            n165 = case shown="\"Enabled\"" w322 {
              tunnel: w323 -> [w330 _]
              frame "Enabled" {
                n166 = property class="DigNum (严格)"(reference=w330) -> (reference out=w327:refnum<vi>, "Value"=w328:sgl)  [unwired: 1 in, 1 out]
                n167 = call "数字键盘.vi"("OldNumber"=w328) -> ("NewNumber"=w329:dbl)  [unwired: 1 in]
                n168 = property class="DigNum (严格)"(reference=w327, "Val(Sgnl)"=w329) -> ()  [unwired: 1 in, 2 out]
              }
              frame "Disabled", Default {
              }
            }
            n169 = call "Add State to Queue.vi"("State(s) In (\"\")"=w324) -> ("States Out"=w325:string)  [unwired: 14 in]
          }
          event "标液1": Value Change {
            n170 = event-data() -> ("NewVal"=w332:sgl)  [unwired: 1 in, 5 out]
            n171 = global read "多参数全局变量.vi" "MB session in"() -> (w333:refnum<class "MB_Master.lvclass">)
            n172 = call "纳清叶绿素a_第一点校准数据写入.vi"("数值"=w332, "MB session in"=w333) -> ()  [unwired: 8 in, 2 out]
            n173 = call "Add State to Queue.vi"("State(s) In (\"\")"=w331) -> ("States Out"=w335:string)  [unwired: 14 in]
          }
          event "标液2": Value Change {
            n174 = event-data() -> ("NewVal"=w337:sgl)  [unwired: 1 in, 5 out]
            n175 = global read "多参数全局变量.vi" "MB session in"() -> (w338:refnum<class "MB_Master.lvclass">)
            n176 = call "纳清叶绿素a_第二点校准数据写入.vi"("数值"=w337, "MB session in"=w338) -> ()  [unwired: 8 in, 2 out]
            n177 = call "Add State to Queue.vi"("State(s) In (\"\")"=w336) -> ("States Out"=w340:string)  [unwired: 14 in]
          }
          event "标液3": Value Change {
            n178 = event-data() -> ("NewVal"=w342:sgl)  [unwired: 1 in, 5 out]
            n179 = global read "多参数全局变量.vi" "MB session in"() -> (w343:refnum<class "MB_Master.lvclass">)
            n180 = call "纳清叶绿素a_第三点校准数据写入.vi"("数值"=w342, "MB session in"=w343) -> ()  [unwired: 8 in, 2 out]
            n181 = call "Add State to Queue.vi"("State(s) In (\"\")"=w341) -> ("States Out"=w345:string)  [unwired: 14 in]
          }
          event "量程": Value Change {
            n182 = event-data() -> ("NewVal"=w347:u16)  [unwired: 1 in, 5 out]
            n183 = global read "多参数全局变量.vi" "MB session in"() -> (w348:refnum<class "MB_Master.lvclass">)
            n184 = call "纳清浊度_量程写入.vi"("数值"=w347, "MB session in"=w348) -> ()  [unwired: 8 in, 2 out]
            n185 = call "Add State to Queue.vi"("State(s) In (\"\")"=w346) -> ("States Out"=w350:string)  [unwired: 14 in]
          }
          event "校准量程": Value Change {
            n186 = event-data() -> ("NewVal"=w352:u16)  [unwired: 1 in, 5 out]
            n187 = global read "多参数全局变量.vi" "MB session in"() -> (w353:refnum<class "MB_Master.lvclass">)
            n188 = call "纳清浊度_校准量程写入.vi"("数值"=w352, "MB session in"=w353) -> ()  [unwired: 8 in, 2 out]
            n189 = call "Add State to Queue.vi"("State(s) In (\"\")"=w351) -> ("States Out"=w355:string)  [unwired: 14 in]
          }
          event "校准启动": Value Change {
            n190 = event-data() -> ()  [unwired: 1 in, 6 out]
            n191 = global read "多参数全局变量.vi" "校准运行状态"() -> (w357:T6)
            n192 = Bundle By Name(cluster=w357, "Turb"=TRUE ("Cond")) -> (w358:T6)
            n193 = global write "多参数全局变量.vi" "校准运行状态"(w358) -> ()
            n194 = call "Add State to Queue.vi"("State(s) In (\"\")"=w362, "State(s) At Back (\"\")"="init: all\nCal: Place standard solution\n Cal: Calibration process\nidle" ("State(s) In (\"\")")) -> ("States Out"=w361:string)  [unwired: 13 in]
          }
          event "校准停止": Value Change {
            n195 = event-data() -> ()  [unwired: 1 in, 6 out]
            n196 = call "Add State to Queue.vi"("State(s) In (\"\")"="init: all\nCal: Over\nidle" ("State(s) In (\"\")")) -> ("States Out"=w364:string)  [unwired: 14 in]
          }
        }
      }
    }
  }
